vi "Drive Straight PID.vi"() -> ()   [LabVIEW 2016]
uses:
  <vilib>/addons/control/pid/pid.llb/PID (DBL).vi
  <vilib>/addons/control/pid/NI_PID_pid.lvlib
panel:
  in  "Reinitialize":bool
  out "Right Power":dbl
  out "Left Power":dbl
  in  "Gyro Angle":dbl
  in  "Current Distance":dbl
  in  "Target Distance":dbl
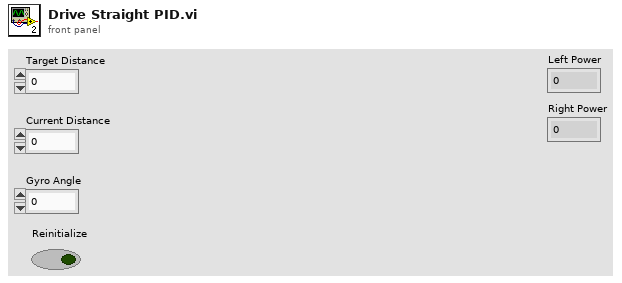
[diagram p1: front panel]
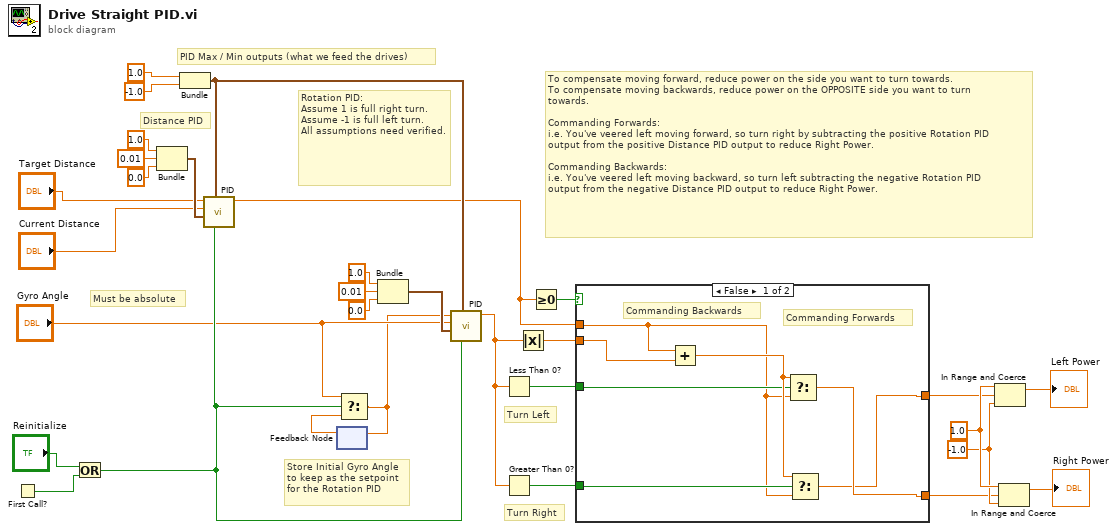
[diagram p0: block diagram]
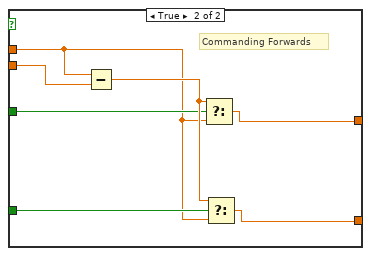
[diagram p2: hidden frame]
diagram:
  w8 = -1.0
  w9 = 1.0
  # "Turn Right"
  # "Turn Left"
  # "To compensate moving forward, reduce power on the side you want to turn towards.\nTo compensate moving backwards, reduce power on the OPPOSITE side you want to turn\ntowards.\n\nCommanding Forwards:\ni.e. You've veered left moving forward, so turn right by subtracting the positive Rotation PID\noutput from the positive Distance PID output to reduce Right Power.\n\nCommanding Backwards:\ni.e. You've veered left moving backward, so turn left subtracting the negative Rotation PID \noutput from the negative Distance PID output to reduce Right Power."
  # "PID Max / Min outputs (what we feed the drives)"
  # "Must be absolute"
  # "Rotation PID:\nAssume 1 is full right turn.\nAssume -1 is full left turn.\nAll assumptions need verified."
  # "Distance PID"
  # "Store Initial Gyro Angle\nto keep as the setpoint\nfor the Rotation PID"
  n1 = First Call?() -> (First Call?: T/F=w22:bool)
  n2 = Or(x="Reinitialize", y=w22) -> (x .or. y?=w16:bool)
  n3 = Bundle(1.0, 0.01, 0.0) -> (w26:cluster{dbl, dbl, dbl})  [unwired: 1 in]
  n4 = Bundle(1.0, -1.0) -> (w17:cluster{dbl, dbl})  [unwired: 1 in]
  n5 = call-poly <vilib>:"PID.vi"("reinitialize? (F)"=w16, "output range"=w17, "PID gains"=w26, "process variable"="Current Distance", "setpoint"="Target Distance") -> ("output"=w7:dbl)  [unwired: 5 in, 1 out]
  n6 = feedback #1() -> (w14:dbl)  [unwired: 1 in]
  n7 = Select(t="Gyro Angle", s=w16, f=w14) -> (s? t:f=w13:dbl)
  n8 = feedback-in #1(w13) -> ()
  n9 = Bundle(1.0, 0.01, 0.0) -> (w18:cluster{dbl, dbl, dbl})  [unwired: 1 in]
  n10 = call-poly <vilib>:"PID.vi"("reinitialize? (F)"=w16, "output range"=w17, "PID gains"=w18, "process variable"="Gyro Angle", "setpoint"=w13) -> ("output"=w3:dbl)  [unwired: 5 in, 1 out]
  n11 = Less Than 0?(x=w3) -> (x < 0?=w2:bool)
  n12 = Greater Than 0?(x=w3) -> (x > 0?=w1:bool)
  n13 = Absolute Value(x=w3) -> (abs(x)=w6:dbl)
  n14 = Greater Or Equal To 0?(x=w7) -> (x >= 0?=w12:bool)
  n15 = case shown="False" w12 {
    tunnel: w6 -> [w35 w45]
    tunnel: w7 -> [w32 w39]
    tunnel: [w34 w43] -> w5
    tunnel: [w33 w42] -> w4
    tunnel: w2 -> [w37 w41]
    tunnel: w1 -> [w36 w40]
    frame False {
      # "Commanding Forwards"
      # "Commanding Backwards"
      n16 = Add(x=w32, y=w35) -> (x+y=w38:dbl)
      n17 = Select(t=w38, s=w37, f=w32) -> (s? t:f=w34:dbl)
      n18 = Select(t=w38, s=w36, f=w32) -> (s? t:f=w33:dbl)
    }
    frame True {
      # "Commanding Forwards"
      n19 = Subtract(x=w39, y=w45) -> (x-y=w44:dbl)
      n20 = Select(t=w44, s=w41, f=w39) -> (s? t:f=w42:dbl)
      n21 = Select(t=w44, s=w40, f=w39) -> (s? t:f=w43:dbl)
    }
  }
  n22 = In Range and Coerce(upper limit=w9, x=w4, lower limit=w8) -> (coerced(x)=→"Left Power":dbl)  [unwired: 1 out]
  n23 = In Range and Coerce(upper limit=w9, x=w5, lower limit=w8) -> (coerced(x)=→"Right Power":dbl)  [unwired: 1 out]
